vi "Volt_to_board_0.vi"(8 "error in (no error)":errorcluster) -> (0 "error out":errorcluster)   [LabVIEW 2015]
doc: "This VI writes the <b>values to write</b> to the <b>addresses</b> for the specified <b>board</b>."
uses:
  <vilib>/Instr/_visa.llb/VISA Register Access Address Space.ctl
panel:
  in  "values to write":u8[](array[numeric]) format="%02d"
  in  "addresses":u32[](array[numeric]) format="%02d"
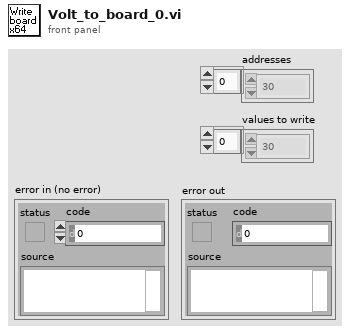
[diagram p1: front panel]
types:
  T1 = typedef "VISA Register Access Address Space.ctl" = u16
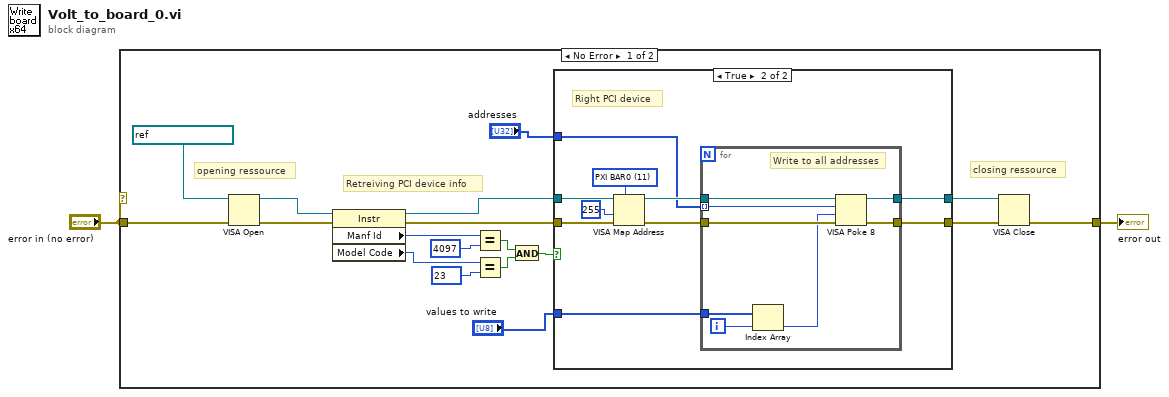
[diagram p0: block diagram]
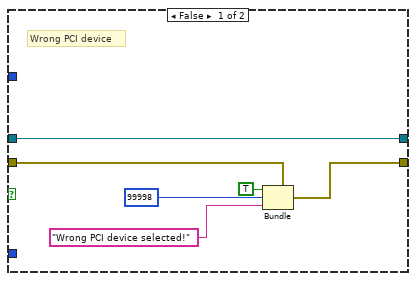
[diagram p2: hidden frame]
diagram:
  n1 = case shown="No Error" "error in (no error)" {
    tunnel: "error in (no error)" -> [w20 w45]
    tunnel: [w10 w45] -> w2
    frame No Error {
      # "closing ressource"
      # "opening ressource"
      # "Retreiving PCI device info"
      n2 = VISA Open(error in (no error)=w20, VISA resource name=refnum<visa-resource-name> "PXI4::5::INSTR" ("board")) -> (VISA resource name=w7:refnum<visa-resource-name>, error out=w19:errorcluster)  [unwired: 3 in]
      n3 = property class="Instr"(reference=w7, error in=w19) -> (reference out=w6:refnum<visa-resource-name>, error out=w14:errorcluster, "Manf Id"=w13:u16, "Model Code"=w12:u16)
      n4 = Equal?(x=w13, y=u16 4097) -> (x = y?=w16:bool)
      n5 = Equal?(x=w12, y=u16 23) -> (x = y?=w17:bool)
      n6 = And(x=w16, y=w17) -> (x .and. y?=w3:bool)
      n7 = case shown="True" w3 {
        tunnel: [w21 w28] -> w9
        tunnel: w6 -> [w21 w30]
        tunnel: w14 -> [w23 w35]
        tunnel: [w22 w36] -> w11
        tunnel: "addresses" -> [_ w27]
        tunnel: "values to write" -> [_ w31]
        frame False {
          # "Wrong PCI device"
          n8 = Bundle(cluster=w23, "status"=TRUE, "code"=99998, "source"="Wrong PCI device selected!") -> (w22:errorcluster)
        }
        frame True {
          w33 = T1 11 items=["VXI/VME A16"=1, "VXI/VME A24"=2, "VXI/VME A32"=3, "VXI/VME A64"=4, "PXI Memory Allocations"=9, "PXI Configuration"=10, "PXI BAR0"=11, "PXI BAR1"=12, "PXI BAR2"=13, "PXI BAR3"=14, "PXI BAR4"=15, "PXI BAR5"=16] ("Address Space")
          # "Right PCI device"
          n9 = VISA Map Address(7:w33, 8:w35, 9:u32 255 ("map size (0)"), 11:w30) -> (0:w34:errorcluster, 3:w29:refnum<visa-resource-name>)  [unwired: 2 in]
          n10 = for {
            tunnel: w29 -> [w37]
            tunnel: [w44] -> w28
            tunnel: w34 -> [w43]
            tunnel: [w42] -> w36
            tunnel: w27 -> [w41] mode=indexing
            tunnel: w31 -> [w39]
            i -> [w38]
            # "Write to all addresses"
            n11 = Index Array(array=w39, index=w38) -> (element=w40:u8)
            n12 = VISA Poke 8(8:w43, 9:w40, 10:w41, 11:w37) -> (0:w42:errorcluster, 3:w44:refnum<visa-resource-name>)
          }
        }
      }
      n13 = VISA Close(VISA resource name=w9, error in (no error)=w11) -> (error out=w10:errorcluster)
    }
    frame Error {
    }
  }
  "error out" <- w2
